vi "Get_Mapping_GBL.vi"() -> (1 "LaserScanangles[]":dbl[](array[numeric]), 2 "LaserScandistance[]":dbl[](array[numeric]), 3 "Current_Position":T1)   [LabVIEW 2017]
uses:
  Ctl/Current_Position.ctl
  Mapping_GBL.vi
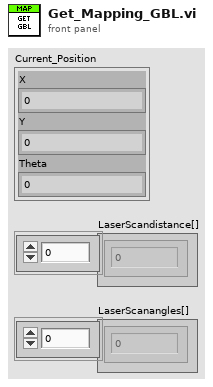
[diagram p1: front panel]
types:
  T1 = typedef "Current_Position.ctl" = cluster{"X":dbl, "Y":dbl, "Theta":dbl}
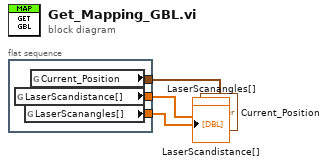
[diagram p0: block diagram]
diagram:
  n1 = flat-sequence {
    tunnel: [w6] -> w1
    tunnel: [w5] -> w2
    tunnel: [w4] -> w3
    frame #0 {
      n2 = global read "Mapping_GBL.vi" "LaserScandistance[]"() -> (w5:dbl[])
      n3 = global read "Mapping_GBL.vi" "LaserScanangles[]"() -> (w4:dbl[])
      n4 = global read "Mapping_GBL.vi" "Current_Position"() -> (w6:T1)
    }
  }
  "LaserScanangles[]" <- w3
  "LaserScandistance[]" <- w2
  "Current_Position" <- w1
